vi "Dashboard Main - Copy (3).vi"() -> ()   [LabVIEW 2014]
uses:
  <vilib>/event_ctls.llb/eventvkey.ctl
  <vilib>/Rock Robotics/WPI/Dashboard/WPI_DashboardLogging Global.vi
  <vilib>/Utility/config.llb/Write Key (String).vi
  <vilib>/Utility/config.llb/Write Key (I32).vi
  <vilib>/Utility/config.llb/NI_LVConfig.lvlib
panel:
  in  "TCP":refnum<k5>
  in  "Rec Mode":enum32{"Stop", "Record", "Playback"}(radio)
  in  "Vision":u16(ring) items=["Camera Off", "USB Camera SW", "USB Camera HW", "IP Camera"]
  out "Camera IP":string
  out "Image Message":string="Timeout in Camera Communications"
  in  "Dashboard Tab":T1(tab)
  out "Low Battery":bool
  out "FMS":bool
  out "Teleop Mode":bool
  out "Auto Mode":bool
  out "Disabled":bool
  in  "Program":string
  in  "Camera Settings":T2={"Frame Rate"=30, "Compression"=30, "Size"=1} {"Frame Rate" scale=1.0..30.0; "Size" items=["640x480", "320x240", "160x120"]}
  out "Mode":T3(ring)=enum."Auto Disabled"
  in  "DB Camera Config":bool
  out "fps":dbl format="%#.1g"
  out "Mbps":dbl format="%#.1g"
  out "Mbps 2":bool
  in  "LCD_Line_10":string caption="DB/String 0"
  in  "LCD_Line_9":string caption="DB/String 0"
  in  "LCD_Line_8":string caption="DB/String 0"
  in  "LCD_Line_7":string caption="DB/String 0"
  in  "LCD_Line_6":string caption="DB/String 0"
  in  "LCD_Line_5":string caption="DB/String 0"
  in  "LCD_Line_4":string caption="DB/String 0"
  in  "LCD_Line_3":string caption="DB/String 0"
  in  "LCD_Line_2":string caption="DB/String 0"
  in  "LCD_Line_1":string caption="DB/String 0"
  in  "DB/String 9":string
  in  "DB/String 8":string
  in  "DB/String 7":string
  in  "DB/String 6":string
  in  "DB/String 5":string
  in  "DB/String 4":string
  in  "DB/String 3":string
  in  "DB/String 2":string
  in  "DB/String 1":string
  in  "DB/String 0":string
  in  "DB/Slider 0":dbl(slide) scale=0.0..5.0
  in  "DB/Slider 1":dbl(slide) scale=0.0..5.0
  in  "DB/Slider 2":dbl(slide) scale=0.0..5.0
  in  "DB/Slider 3":dbl(slide) scale=0.0..5.0
  out "DB/LED 3":bool
  out "DB/LED 2":bool
  out "DB/LED 1":bool
  out "DB/LED 0":bool
  in  "DB/Button 3":bool
  in  "DB/Button 2":bool
  in  "DB/Button 1":bool
  in  "DB/Button 0":bool caption="New Name"
  in  "Test Slider":dbl(slide) scale=0.0..100.0 scale format="%#_3g"
  in  "On/Off":bool caption="Solenoid"
  in  "Test Name":u16(ring) items=["Select the test to run...", "Example Test", "-------------------------------", "List of tests is built in robot code.", "Replace with your own automated tests."]
  in  "Test Tree":string(tree)
  in  "Motor":cluster{"Value":dbl, "Enable":bool} {"Value" scale=-1.0..1.0 scale format="%#_3g"}
  out "Progress":T4 {"Test Progress" scale=0.0..100.0}
  in  "Rev/Fwd":cluster{"Forward":bool, "Reverse":bool}
  in  "Test Ring":u16(ring) items=["Monochrome", "Color"]
  in  "Listbox":i32(listbox)
  out "Tree":string(tree)
  out "Camera Image":T5(plugin-control)
  out "Boolean":bool
  # "Program:"
  # "Dashboard: 2015-02"
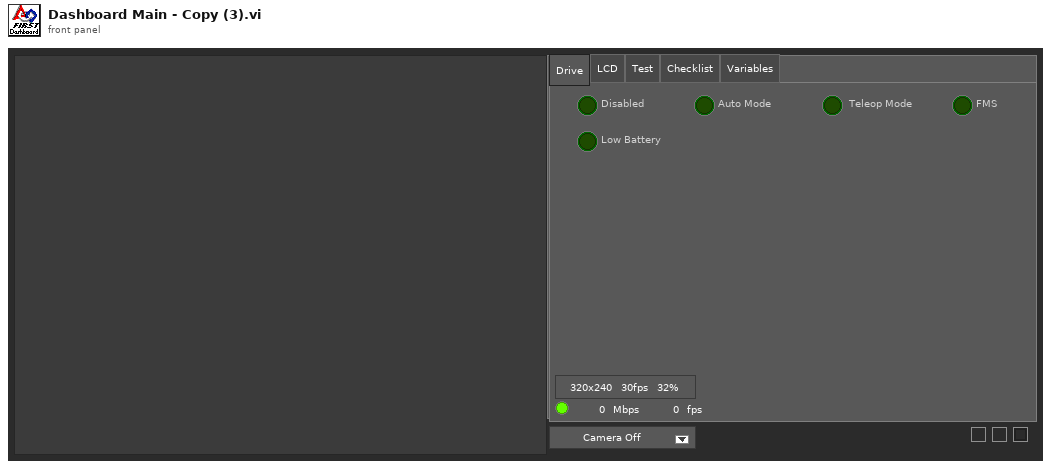
[diagram p1: front panel]
types:
  T1 = enum32{"Drive", "LCD", "Basic", "Test", "Checklist", "Variables"}
  T2 = cluster{"Frame Rate":i32, "Compression":i32, "Size":u16}
  T3 = enum8{"Tele-Op Disabled", "Tele-Op Enabled", "Auto Disabled", "Auto Enabled", "Test Disabled", "Test Enabled", "Disconnected", "No Code", "E-Stop"}
  T4 = cluster{"Test Progress":u8, "Test Progress Text":string}
  T5 = typedef "IMAQ Image.ctl" = refnum<image>
  T6 = enum32{"Drive", "Basic", "Custom", "Test", "Checklist", "Variables"}
  T7 = typedef "Image Type" = u32
  T8 = cluster{"Camera Image":refnum<vi>, "Dashboard Tab":refnum<vi>, "Boolean":refnum<vi>, "Vision":refnum<vi>, "Rec Mode":refnum<vi>, "Test Slider":refnum<vi>, "On/Off ":refnum<vi>, "Test Ring":refnum<vi>, "Rev/Fwd":refnum<vi>, "Test Name":refnum<vi>, "Motor":refnum<vi>, "Progress":refnum<vi>, "CheckList":refnum<vi>, "Tree":refnum<vi>, "Test Tree":refnum<vi>}
  T9 = cluster{"Error Strings":string, "Disable Counts":cluster{u16, u16}, "Rail Faults":cluster{u16, u16, u16}, "Robot IP":string, "DB Mode":u8, "Event Info":cluster{"Name":string, "Type":u8, "Number":u16, "Replay":u8}, "Camera Addr":string}
  T10 = cluster{"Storage":cluster{"Disk Free":u64, "RAM Block":u32, "RAM free":u32}, "CPU Utilization":cluster{"CPU % ISR":sgl, "CPU % Time Crit":sgl, "CPU % Timed Str":sgl, "CPU % High":sgl, "CPU % Above":sgl, "CPU % Normal":sgl, "CPU % Low":sgl}, "CAN":cluster{"% Bus Utilization":sgl, "Bus Off Cnt":u32, "TX_FIFO Full Cnt":u32, "Receive Error Cnt":u8, "Transmit Error Cnt":u8}, "HID":cluster{"HID Outputs":u32, "Rumble Low":u16, "Rumble High":u16}[]}
  T11 = cluster{"Status bits":cluster{"Test Mode":bool, "Autonomous":bool, "Enabled":bool, "Code Start":bool, "Brownout":bool, "Reserved 2":bool, "Reserved 3":bool, "E-Stop":bool}, "Code Trace":cluster{"Disabled":bool, "TeleOp":bool, "Auto":bool, "Test":bool}, "Controller Type":enum16{"unknown", "cRIO", "roboRio"}, "Code?":enum16{"unknown", "noCode", "code"}, "Battery V":dbl}
  T12 = cluster{"Control Bits":cluster{"TestMode":bool, "Autonomous":bool, "Enabled":bool, "FMS Present":bool, bool, bool, bool, "E-Stop":bool}, "Team Station ":u8, "Countdown":sgl, "Joystick Values":cluster{"Axes":dbl[], "Buttons":bool[], "POVs":i16[]}[]}
  T13 = cluster{"Axes":dbl[], "Buttons":bool[], "POVs":i16[]}[]
  T14 = cluster{"Axes":dbl[], "Buttons":bool[], "POVs":i16[]}
  T15 = typedef "NI_LVConfig.lvlib/Config Data RefNum.ctl" = refnum<k1>
  T16 = cluster{"Operation":enum16{"Update", "Clear"}, "Color Box":u32}[]
  T17 = typedef "eventvkey.ctl" = enum16{"ASCII", "Enter", "Return", "Shift", "Ctrl", "Alt", "Cmd", "Opt", "Caps", "NumLock", "Clear", "Break", "Up", "Down", "Left", "Right", "Insert", "Delete", "Home", "End", "PageUp", "PageDown", "Escape", "Help", "Pause", "ScrollLock", "F1", "F2", "F3", "F4", "F5", "F6", "F7", "F8", "F9", "F10", "F11", "F12", "F13", "F14", "F15", "F16", "F17", "F18", "F19", "F20", "F21", "F22", "F23", "F24", "Play", "VolumeUp", "VolumeDown", "Mute", "Two Byte Char"}
  T18 = cluster{"Image Size":bool, "Image Type":bool, "Pixel Value":bool, "ROI Information":bool, "Zoom Factor":bool}
  T19 = enum8{"Enabled", "Disabled", "Disabled and Grayed Out"}
  T20 = cluster{"Operation":enum16{"Update", "Clear"}, "Color Box":u32}
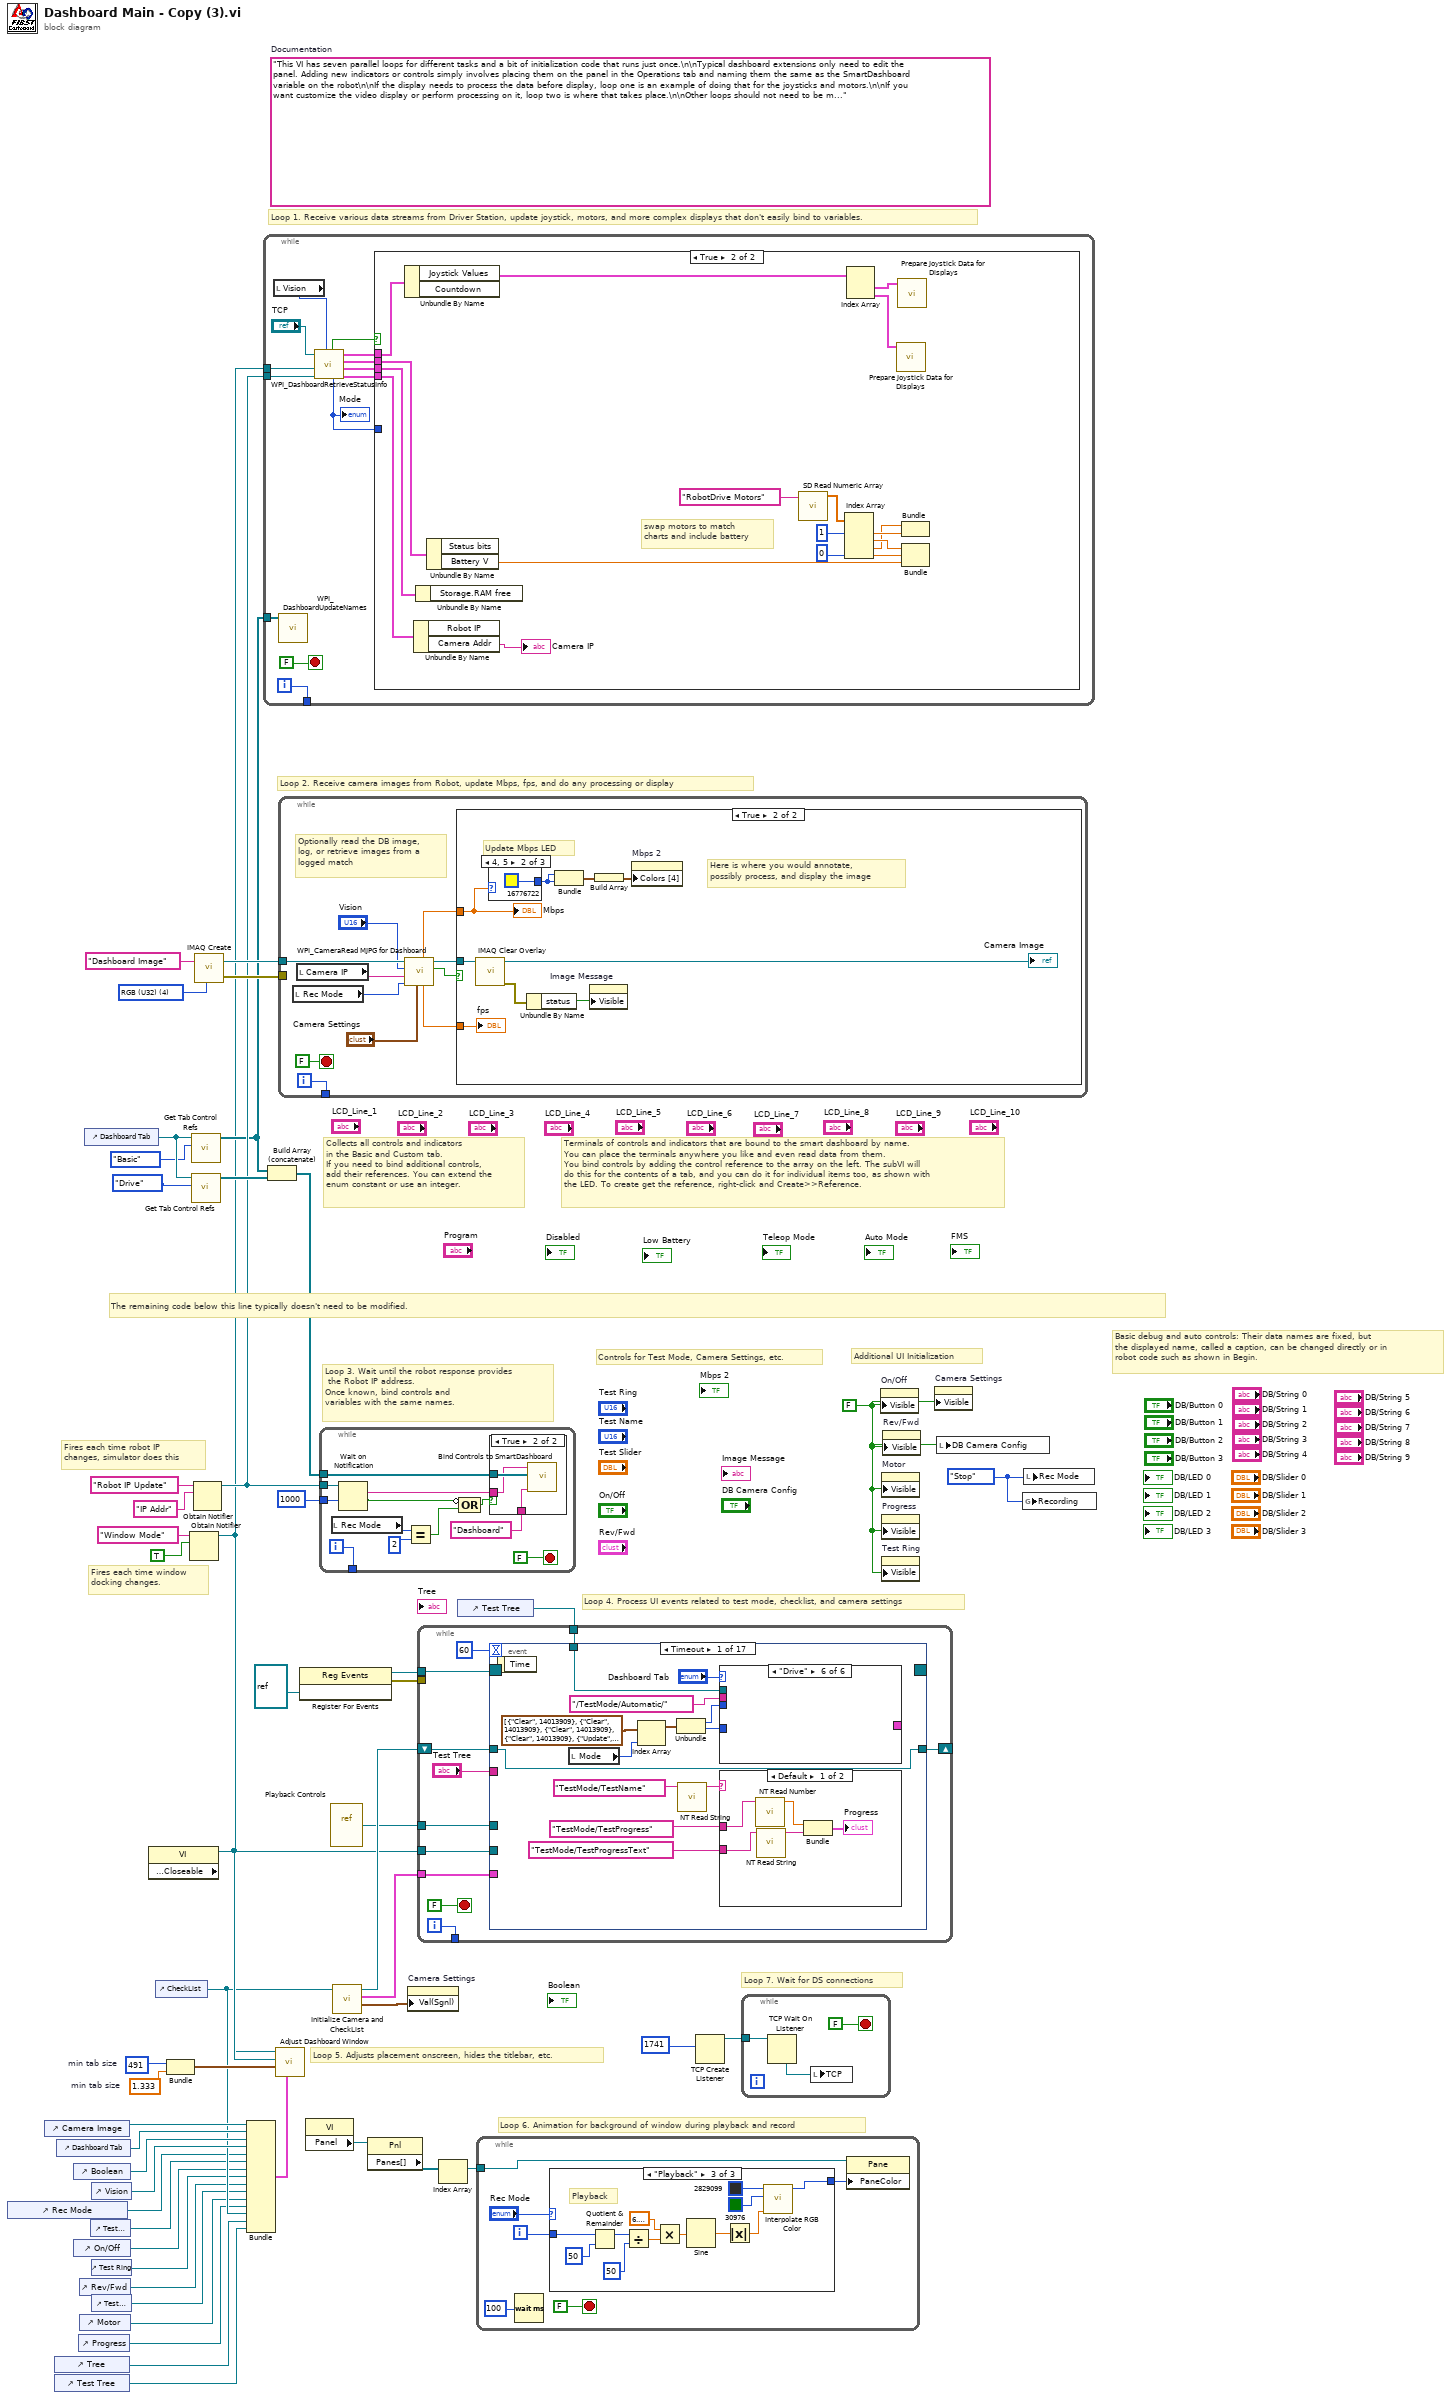
[diagram p0: block diagram]
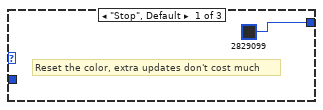
[diagram p3: hidden frame]
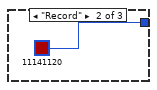
[diagram p4: hidden frame]
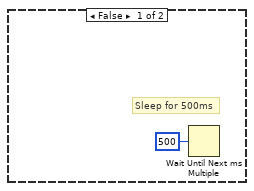
[diagram p6: hidden frame]
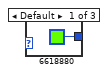
[diagram p7: hidden frame]
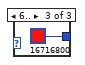
[diagram p8: hidden frame]
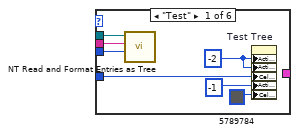
[diagram p9: hidden frame]
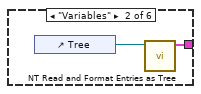
[diagram p10: hidden frame]
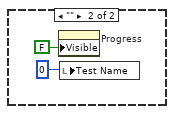
[diagram p14: hidden frame]
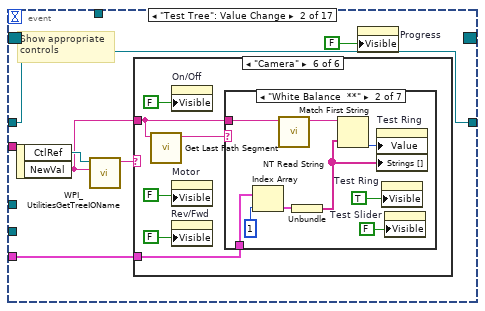
[diagram p15: hidden frame]
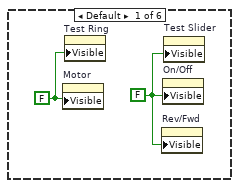
[diagram p16: hidden frame]
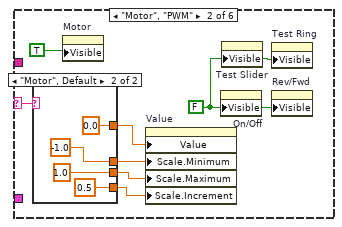
[diagram p17: hidden frame]
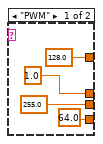
[diagram p18: hidden frame]
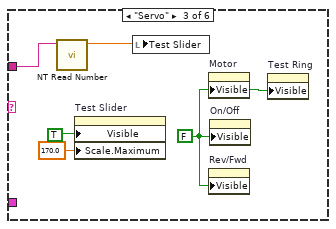
[diagram p19: hidden frame]
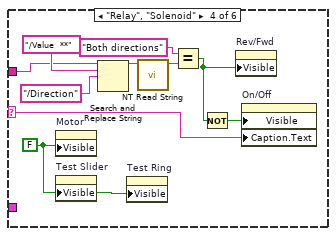
[diagram p20: hidden frame]
diagram:
  w24 = 491  # min tab size
  w23 = 1.333  # min tab size
  w32 = enum32{"Stop", "Record", "Playback"}."Stop" ("Rec Mode")
  w6 = FALSE ("Visible")
  (unwired) "This VI has seven parallel loops for different tasks and a bit of initialization code that runs just once.\n\nTypical dashboard extensions only need to edit the panel. Adding new indicators or controls simply involves placing them on the panel in the Operations tab and naming them the same as the SmartDashboard variable on the robot\n\nIf the display needs to process the data before display, loop one is an example of doing that for the joysticks and motors.\n\nIf you want customize the video display or perform processing on it, loop two is where that takes place.\n\nOther loops should not need to be modified. They are pretty standard, and document the task they perform."  # Documentation
  w52 = T7 4 items=["Grayscale (U8)", "Grayscale (I16)", "Grayscale (SGL)", "Complex (CSG)", "RGB (U32)", "HSL (U32)", "RGB (U64)"] ("Image Type")
  # "Loop 7. Wait for DS connections"
  # "Basic debug and auto controls: Their data names are fixed, but\nthe displayed name, called a caption, can be changed directly or in\nrobot code such as shown in Begin."
  # "Controls for Test Mode, Camera Settings, etc."
  # "Additional UI Initialization"
  # "Loop 6. Animation for background of window during playback and record"
  # "Fires each time robot IP\nchanges, simulator does this"
  # "Fires each time window\ndocking changes."
  # "Collects all controls and indicators\nin the Basic and Custom tab.\nIf you need to bind additional controls,\nadd their references. You can extend the\nenum constant or use an integer."
  # "The remaining code below this line typically doesn't need to be modified."
  # "Loop 4. Process UI events related to test mode, checklist, and camera settings"
  # "Terminals of controls and indicators that are bound to the smart dashboard by name.\nYou can place the terminals anywhere you like and even read data from them.\nYou bind controls by adding the control reference to the array on the left. The subVI will\ndo this for the contents of a tab, and you can do it for individual items too, as shown with\nthe LED. To create get the reference, right-click and Create>>Reference."
  # "Loop 3. Wait until the robot response provides\n the Robot IP address.\nOnce known, bind controls and\nvariables with the same names."
  # "Loop 5. Adjusts placement onscreen, hides the titlebar, etc."
  # "Loop 1. Receive various data streams from Driver Station, update joystick, motors, and more complex displays that don't easily bind to variables."
  # "Loop 2. Receive camera images from Robot, update Mbps, fps, and do any processing or display"
  n1 = control-ref of="Rec Mode"() -> (w12:refnum<vi>)
  n2 = control-ref of="Camera Image"() -> (w27:refnum<vi>)
  n3 = control-ref of="Tree"() -> (w16:refnum<vi>)
  n4 = control-ref of="Test Tree"() -> (w15:refnum<vi>)
  n5 = control-ref of="Dashboard Tab"() -> (w26:refnum<vi>)
  n6 = control-ref of="Boolean"() -> (w21:refnum<vi>)
  n7 = control-ref of="On/Off"() -> (w10:refnum<vi>)
  n8 = control-ref of="Progress"() -> (w7:refnum<vi>)
  n9 = control-ref of="Rev/Fwd"() -> (w8:refnum<vi>)
  n10 = control-ref of="Motor"() -> (w13:refnum<vi>)
  n11 = control-ref of="Dashboard Tab"() -> (w30:refnum<vi>)
  n12 = control-ref of="Test Slider"() -> (w11:refnum<vi>)
  n13 = control-ref of="Vision"() -> (w25:refnum<vi>)
  n14 = control-ref of="Test Ring"() -> (w9:refnum<vi>)
  n15 = control-ref of="Test Name"() -> (w14:refnum<vi>)
  n16 = property class="VI" props=["Front Panel.Closeable"]() -> (reference out=w31:refnum<vi>)  [unwired: 2 in, 2 out]
  n17 = control-ref of="CheckList"() -> (w17:refnum<vi>)
  n18 = Bundle("min tab size"=w24, "min tab size"=w23) -> (w22:cluster{"min tab size":i32, "min tab size":dbl})  [unwired: 1 in]
  n19 = Obtain Notifier(name (unnamed)="Window Mode", notification data type=TRUE) -> (notifier out=w3:refnum<notifier>)  [unwired: 2 in, 2 out]
  n20 = call <vilib>:"Get Tab Control Refs.vi"("Page Index"=T6."Basic" ("Dashboard Tab"), "TabControl in"=w30) -> ("ControlsOnPage"=w4:refnum<vi>[])  [unwired: 9 in]
  n21 = call <vilib>:"Get Tab Control Refs.vi"("Page Index"=T6."Drive" ("Dashboard Tab"), "TabControl in"=w30) -> ("ControlsOnPage"=w29:refnum<vi>[])  [unwired: 9 in]
  n22 = Obtain Notifier(name (unnamed)="Robot IP Update", notification data type="IP Addr" ("name (unnamed)")) -> (notifier out=w5:refnum<notifier>)  [unwired: 2 in, 2 out]
  n23 = call "IMAQ Create"("Image Name"="Dashboard Image", "Image Type"=w52) -> ("New Image"=w50:T5, "error out"=w49:errorcluster)  [unwired: 2 in, 1 out]
  n24 = Bundle("Camera Image"=w27, "Dashboard Tab"=w26, "Boolean"=w21, "Vision"=w25, "Rec Mode"=w12, "Test Slider"=w11, "On/Off"=w10, "Test Ring"=w9, "Rev/Fwd"=w8, "Test Name"=w14, "Motor"=w13, "Progress"=w7, "CheckList"=w17, "Tree"=w16, "Test Tree"=w15) -> (w18:T8)  [unwired: 1 in]
  n25 = while {
    tunnel: [w64] -> _
    tunnel: w5 -> [w58]
    tunnel: w4 -> [w57]
    tunnel: w3 -> [w53]
    i -> [w64]
    stop <- FALSE stop-if-true
    n26 = local read "Vision"() -> (w55:u16)
    n27 = call <vilib>:"WPI_DashboardUpdateNames.vi"("Controls on Tab"=w57) -> ()  [unwired: 11 in]
    n28 = call <vilib>:"WPI_DashboardRetrieveStatusInfo.vi"("Vision"=w55, "Binding Refnum"=w58, "Window Mode Notifier"=w53, "TCP Cnx"="TCP") -> ("Power and Errors"=w59:T9, "Robot Metrics"=w62:T10, "Status Info"=w63:T11, "Control Info"=w60:T12, "Robot Mode"=w56:T3, "Process?"=w61:bool)  [unwired: 2 in]
    "Mode" <- w56
    n29 = case shown="True" w61 {
      tunnel: w63 -> [_ w82]
      tunnel: w62 -> [_ w81]
      tunnel: w60 -> [_ w80]
      tunnel: w59 -> [_ w79]
      tunnel: w56 -> [_ _]
      frame False {
      }
      frame True {
        # "swap motors to match\ncharts and include battery"
        n30 = Unbundle By Name(w80) -> ("Joystick Values"=w69:T13)  [unwired: 1 out]
        n31 = Unbundle By Name(w79) -> ("Camera Addr"=→"Camera IP":string)  [unwired: 1 out]
        n32 = Unbundle By Name(w81) -> ()  [unwired: 1 out]
        n33 = Unbundle By Name(w82) -> ("Battery V"=w70:dbl)  [unwired: 1 out]
        n34 = call <vilib>:"SD Read Numeric Array.vi"("Name"="RobotDrive Motors") -> ("Numeric Array"=w72:dbl[])  [unwired: 8 in, 2 out]
        n35 = Index Array(array=w72, index #1=1, index #4=0) -> (element #1=w74:dbl, element #2=w75:dbl, element #3=w73:dbl, element #4=w78:dbl)  [unwired: 2 in]
        n36 = Index Array(array=w69) -> (element #1=w68:T14, element #2=w66:T14)  [unwired: 2 in]
        n37 = call "Prepare Joystick Data for Displays.vi"("Joystick Values"=w66) -> ()  [unwired: 8 in, 3 out]
        n38 = call "Prepare Joystick Data for Displays.vi"("Joystick Values"=w68) -> ()  [unwired: 8 in, 3 out]
        n39 = Bundle("Numeric"=w73, "Numeric"=w74) -> ()  [unwired: 1 in, 1 out]
        n40 = Bundle("Numeric"=w75, "Numeric"=w78, "Battery V"=w70) -> ()  [unwired: 1 in, 1 out]
      }
    }
  }
  n41 = Build Array (concatenate)(w4, w29) -> (w28:refnum<vi>[])
  n42 = call "Adjust Dashboard Window.vi"("Sizing Refnums"=w18, "Size Constraints"=w22, "VI"=w31, "Notifier in"=w3) -> ()  [unwired: 8 in]
  n43 = while {
    tunnel: w50 -> [w91]
    tunnel: w49 -> [_]
    tunnel: [w92] -> _
    i -> [w92]
    stop <- FALSE stop-if-true
    # "Optionally read the DB image,\nlog, or retrieve images from a\nlogged match"
    n44 = local read "Rec Mode"() -> (w85:enum32{"Stop", "Record", "Playback"})
    n45 = local read "Camera IP"() -> (w83:string)
    n46 = call <vilib>:"WPI_CameraRead MJPG for Dashboard.vi"("Camera Settings"="Camera Settings", "Rec Mode"=w85, "Camera IP"=w83, "Camera Mode"="Vision", "Refnum in"=w91) -> ("Active"=w89:bool, "Refnum out"=w90:T5, "FPS"=w88:dbl, "Bandwidth (Mbps)"=w87:dbl)  [unwired: 3 in]
    n47 = case shown="True" w89 {
      tunnel: w90 -> [_ w98]
      tunnel: w87 -> [_ w97]
      tunnel: w88 -> [_ w95]
      frame False {
        # "Sleep for 500ms"
        n48 = Wait Until Next ms Multiple(millisecond multiple=u32 500) -> ()  [unwired: 1 out]
      }
      frame True {
        # "Here is where you would annotate,\npossibly process, and display the image"
        # "Update Mbps LED"
        n49 = call "IMAQ Clear Overlay"("Image"=w98) -> ("error out"=w102:errorcluster, "Image Out"=→"Camera Image":T5)  [unwired: 2 in, 7 out]
        n50 = case shown="4, 5" w97 {
          tunnel: [u32 6618880 ("Color Box") u32 16776722 ("Color Box") u32 16716800 ("Color Box")] -> w99
          frame Default {
          }
          frame 4, 5 {
          }
          frame 6.. {
          }
        }
        n51 = Unbundle By Name(w102) -> ("status"=w103:bool)
        n52 = Bundle("Color Box"=w99, "Color Box"=w99) -> (w101:cluster{"Color Box":u32, "Color Box":u32})  [unwired: 1 out]
        n53 = property on="Image Message" class="Str"("Visible"=w103) -> ()  [unwired: 2 in, 2 out]
        n54 = Build Array(w101) -> (w100:cluster{"Color Box":u32, "Color Box":u32}[])
        n55 = property on="Mbps 2" class="Bool (strict)"("Colors [4]"=w100) -> ()  [unwired: 2 in, 2 out]
        "Mbps" <- w97
        "fps" <- w95
      }
    }
  }
  n56 = register-events(refnum<vi> refnum) -> (reference out=w36:refnum<event-registration>, error out=w35:errorcluster)  [unwired: 2 in]
  n57 = property class="VI"() -> ("Panel"=w39:refnum<vi>)  [unwired: 2 in, 2 out]
  n58 = while {
    tunnel: w28 -> [w118]
    tunnel: w5 -> [w116]
    tunnel: [w114] -> _
    tunnel: u32 1000 ("milliseconds to wait") -> [w113]
    i -> [w114]
    stop <- FALSE stop-if-true
    n59 = local read "Rec Mode"() -> (w109:enum32{"Stop", "Record", "Playback"})
    n60 = Wait on Notification(notifier=w116, timeout in ms (-1)=w113) -> (notification=w115:string, timed out?=w111:bool)  [unwired: 2 in, 2 out]
    n61 = Equal?(x=w109, y=u16 2 ("Rec Mode")) -> (x = y?=w110:bool)
    n62 = Compound Arithmetic op=OR(invert w111, w110) -> (w112:bool)
    n63 = case shown="True" w112 {
      tunnel: w118 -> [_ w121]
      tunnel: w115 -> [_ w120]
      tunnel: "Dashboard" -> [_ w119]
      frame False {
      }
      frame True {
        n64 = call <vilib>:"Bind Controls to SmartDashboard.vi"("Client Name"=w119, "Bound Control Refs"=w121, "Server IP Address"=w120) -> ()  [unwired: 9 in]
      }
    }
  }
  n65 = vi-ref "Playback Controls.vi"() -> (w37:refnum<vi>)
  n66 = call "Initialize Camera and CheckList.vi"("ListBox in"=w17) -> ("Cluster"=w43:cluster{"value":i32, "value":i32, "index":i32}, "Array"=w44:cluster{string[]}[], "File Refnum"=w42:T15)  [unwired: 8 in]
  n67 = property class="Pnl"(reference=w39) -> ("Panes[]"=w40:refnum<vi>[])  [unwired: 1 in, 2 out]
  n68 = property on="Camera Settings" class="Clust (strict)"("Val(Sgnl)"=w43) -> ()  [unwired: 2 in, 2 out]
  n69 = Index Array(array=w40) -> (element=w38:refnum<vi>)  [unwired: 1 in]
  n70 = control-ref of="Test Tree"() -> (w41:refnum<vi>)
  n71 = while {
    tunnel: w44 -> [w129]
    shift-right: [w128] -> _
    shift-left: w42 -> [w127]
    tunnel: [w126] -> _
    tunnel: w41 -> [w125]
    tunnel: w37 -> [w124]
    tunnel: w36 -> [w123]
    tunnel: w35 -> [_]
    tunnel: w31 -> [w122]
    i -> [w126]
    stop <- FALSE stop-if-true
    n72 = event shown="[0] Timeout" {
      selector: w123 -> [_ _ _ _ _ _ _ _ _ _ _ _ _ _ _ _ _]
      dyn-events: [_ _ _ _ _ _ _ _ _ _ _ _ _ w367 _ _ _] -> _
      timeout: u32 60 ("milliseconds to wait") -> [_ _ _ _ _ _ _ _ _ _ _ _ _ _ _ _ _]
      tunnel: w125 -> [w141 _ _ _ _ _ _ _ _ _ _ _ _ _ _ _ _]
      tunnel: "Test Tree" -> [_ _ _ _ _ _ _ _ w336 w344 w346 w350 w358 _ _ _ _]
      tunnel: w129 -> [_ w163 _ _ _ _ w300 w330 _ _ _ _ _ _ _ _ _]
      tunnel: [w137 w162 w261 w266 w274 w286 w299 w323 w335 w342 w345 w349 w357 w369 w383 w384 w394] -> w128
      tunnel: w127 -> [w137 w162 w261 w266 w274 w286 w298 w323 w335 w342 w345 w349 w357 w369 w383 w384 w394]
      tunnel: w124 -> [_ _ _ _ _ _ _ _ _ _ _ _ _ w370 _ w387 _]
      tunnel: w122 -> [_ _ _ _ _ _ _ _ _ _ _ _ _ w365 _ _ _]
      event Timeout {
        n73 = event-data() -> ()  [unwired: 1 in, 1 out]
        n74 = local read "Mode"() -> (w140:T3)
        n75 = Index Array(array=T16 [{"Operation"=enum."Clear", "Color Box"=14013909}, {"Operation"=enum."Clear", "Color Box"=14013909}, {"Operation"=enum."Clear", "Color Box"=14013909}, {"Operation"=enum."Clear", "Color Box"=14013909}, {"Operation"=enum."Update", "Color Box"=14013909}, {"Operation"=enum."Update", "Color Box"=16777215}, {"Operation"=enum."Clear", "Color Box"=14013909}, {"Operation"=enum."Clear", "Color Box"=14013909}, {"Operation"=enum."Clear", "Color Box"=14013909}], index=w140) -> (element=w135:T20)
        n76 = Unbundle(w135) -> ("Operation"=w134:enum16{"Update", "Clear"}, "Color Box"=w133:u32)
        n77 = call <vilib>:"NT Read String.vi"("Name"="TestMode/TestName") -> ("String"=w144:string)  [unwired: 9 in, 1 out]
        n78 = case shown="\"Drive\"" "Dashboard Tab" {
          tunnel: w141 -> [w152 _ _ _ _ _]
          tunnel: "/TestMode/Automatic/" ("Name Pattern") -> [w151 _ _ _ _ _]
          tunnel: w134 -> [w150 _ _ _ _ _]
          tunnel: [_ w154 _ _ _ _] -> _
          tunnel: w133 -> [w146 _ _ _ _ _]
          frame "Test" {
            w149 = -2 ("Active Item:Row Number")
            n79 = call <vilib>:"NT Read and Format Entries as Tree.vi"("Operation"=w150, "Name Pattern"=w151, "Tree Refnum"=w152) -> ()  [unwired: 7 in, 2 out]
            n80 = property on="Test Tree" class="Tree (strict)"("Active Item Row Number"=w149, "ActiveColNum"=w149, "CellBG"=w146, "Active Item Row Number"=-1 ("Active Item:Row Number"), "CellBG"=u32 5789784 ("Color Box")) -> ()  [unwired: 2 in, 2 out]
          }
          frame "Variables" {
            n81 = control-ref of="Tree"() -> (w153:refnum<vi>)
            n82 = call <vilib>:"NT Read and Format Entries as Tree.vi"("Tree Refnum"=w153) -> ("Formatted Strings"=w154:cluster{"Name":string, "Value":string}[])  [unwired: 9 in, 1 out]
          }
          frame "Checklist" {
          }
          frame "Basic" {
          }
          frame "LCD" {
          }
          frame "Drive" {
          }
        }
        n83 = case shown="Default" w144 {
          tunnel: "TestMode/TestProgress" ("Name") -> [w156 _]
          tunnel: "TestMode/TestProgressText" ("Name") -> [w155 _]
          frame Default {
            n84 = call <vilib>:"NT Read Number.vi"("Name"=w156) -> ("Numeric"=w157:dbl)  [unwired: 9 in, 1 out]
            n85 = call <vilib>:"NT Read String.vi"("Name"=w155) -> ("String"=w158:string)  [unwired: 9 in, 1 out]
            n86 = Bundle("Numeric"=w157, "String"=w158) -> (→"Progress":cluster{"Numeric":dbl, "String":string})  [unwired: 1 in]
          }
          frame "" {
            n87 = property on="Progress" class="Clust (strict)"("Visible"=FALSE) -> ()  [unwired: 2 in, 2 out]
            n88 = local write "Test Name"(u16 0) -> ()
          }
        }
      }
      event "Test Tree": Value Change {
        # "Show appropriate\ncontrols"
        n89 = event-data() -> ("CtlRef"=w166:refnum<vi>, "NewVal"=w164:string)  [unwired: 1 in]
        n90 = call <vilib>:"WPI_UtilitiesGetTreeIOName.vi"("NewVal"=w164, "TreeControl in"=w166) -> ("I/O Name"=w167:string)  [unwired: 9 in]
        n91 = case shown="\"Camera\"" w167 {
          selector: w167 -> [_ w174 _ w192 w201 _]
          tunnel: w164 -> [_ _ w189 w191 _ w208]
          tunnel: w163 -> [_ _ _ _ _ w207]
          frame Default {
            w169 = FALSE ("Visible")
            w168 = FALSE ("Visible")
            n92 = property on="Motor" class="Clust (strict)"("Visible"=w168) -> ()  [unwired: 2 in, 2 out]
            n93 = property on="Test Ring" class="Ring (strict)"("Visible"=w168) -> ()  [unwired: 2 in, 2 out]
            n94 = property on="Rev/Fwd" class="Clust (strict)"("Visible"=w169) -> ()  [unwired: 2 in, 2 out]
            n95 = property on="On/Off" class="Bool (strict)"("Visible"=w169) -> ()  [unwired: 2 in, 2 out]
            n96 = property on="Test Slider" class="Slide (strict)"("Visible"=w169) -> ()  [unwired: 2 in, 2 out]
          }
          frame "Motor", "PWM" {
            w175 = FALSE ("Visible")
            n97 = case shown="\"Motor\", Default" w174 {
              tunnel: [1.0 ("Value") -1.0 ("Value")] -> w173
              tunnel: [255.0 ("Value") 1.0 ("Value")] -> w172
              tunnel: [128.0 ("Value") 0.0 ("Value")] -> w171
              tunnel: [64.0 ("Value") 0.5 ("Value")] -> w170
              frame "PWM" {
              }
              frame "Motor", Default {
              }
            }
            n98 = property on="Motor" class="Clust (strict)"("Visible"=TRUE) -> ()  [unwired: 2 in, 2 out]
            n99 = property on="Value" class="Slide (strict)"("Value"=w171, "Scale.Minimum"=w173, "Scale.Maximum"=w172, "Scale.Increment"=w170) -> ()  [unwired: 2 in, 2 out]
            n100 = property on="On/Off" class="Bool (strict)"("Visible"=w175) -> ()  [unwired: 2 in, 2 out]
            n101 = property on="Test Slider" class="Slide (strict)"("Visible"=w175) -> ()  [unwired: 2 in, 2 out]
            n102 = property on="Test Ring" class="Ring (strict)"("Visible"=w175) -> ()  [unwired: 2 in, 2 out]
            n103 = property on="Rev/Fwd" class="Clust (strict)"("Visible"=w175) -> ()  [unwired: 2 in, 2 out]
          }
          frame "Servo" {
            w187 = FALSE ("Visible")
            n104 = call <vilib>:"NT Read Number.vi"("Name"=w189) -> ("Numeric"=w188:dbl)  [unwired: 9 in, 1 out]
            n105 = property on="Test Slider" class="Slide (strict)"("Visible"=TRUE, "Scale.Maximum"=170.0 ("Scale.Range:Maximum")) -> ()  [unwired: 2 in, 2 out]
            n106 = local write "Test Slider"(w188) -> ()
            n107 = property on="Motor" class="Clust (strict)"("Visible"=w187) -> ()  [unwired: 2 in, 2 out]
            n108 = property on="Rev/Fwd" class="Clust (strict)"("Visible"=w187) -> ()  [unwired: 2 in, 2 out]
            n109 = property on="On/Off" class="Bool (strict)"("Visible"=w187) -> ()  [unwired: 2 in, 2 out]
            n110 = property on="Test Ring" class="Ring (strict)"("Visible"=w187) -> ()  [unwired: 2 in, 2 out]
          }
          frame "Relay", "Solenoid" {
            w190 = FALSE ("Visible")
            n111 = property on="Motor" class="Clust (strict)"("Visible"=w190) -> ()  [unwired: 2 in, 2 out]
            n112 = property on="Test Slider" class="Slide (strict)"("Visible"=w190) -> ()  [unwired: 2 in, 2 out]
            n113 = Search and Replace String(input string=w191, search string="/Value  **", replace string="/Direction") -> (result string=w197:string)  [unwired: 5 in, 3 out]
            n114 = property on="Test Ring" class="Ring (strict)"("Visible"=w190) -> ()  [unwired: 2 in, 2 out]
            n115 = call <vilib>:"NT Read String.vi"("Name"=w197) -> ("String"=w195:string)  [unwired: 9 in, 1 out]
            n116 = Equal?(x="Both directions", y=w195) -> (x = y?=w193:bool)
            n117 = Not(x=w193) -> (.not. x?=w194:bool)
            n118 = property on="Rev/Fwd" class="Clust (strict)"("Visible"=w193) -> ()  [unwired: 2 in, 2 out]
            n119 = property on="On/Off" class="Bool (strict)"("Visible"=w194, "Caption.Text"=w192) -> ()  [unwired: 2 in, 2 out]
          }
          frame "Compressor", "Digital Out" {
            w200 = FALSE ("Visible")
            # "Get direction and finish"
            n120 = property on="Motor" class="Clust (strict)"("Visible"=w200) -> ()  [unwired: 2 in, 2 out]
            n121 = property on="Test Slider" class="Slide (strict)"("Visible"=w200) -> ()  [unwired: 2 in, 2 out]
            n122 = property on="Test Ring" class="Ring (strict)"("Visible"=w200) -> ()  [unwired: 2 in, 2 out]
            n123 = property on="On/Off" class="Bool (strict)"("Visible"=TRUE, "Caption.Text"=w201) -> ()  [unwired: 2 in, 2 out]
            n124 = property on="Rev/Fwd" class="Clust (strict)"("Visible"=FALSE) -> ()  [unwired: 2 in, 2 out]
          }
          frame "Camera" {
            n125 = call <vilib>:"Get Last Path Segment.vi"("String in"=w208) -> ("String out"=w209:string)  [unwired: 10 in]
            n126 = property on="On/Off" class="Bool (strict)"("Visible"=FALSE) -> ()  [unwired: 2 in, 2 out]
            n127 = property on="Motor" class="Clust (strict)"("Visible"=FALSE) -> ()  [unwired: 2 in, 2 out]
            n128 = property on="Rev/Fwd" class="Clust (strict)"("Visible"=FALSE) -> ()  [unwired: 2 in, 2 out]
            n129 = case shown="\"White Balance  **\"" w209 {
              tunnel: w208 -> [w215 w224 w233 w242 w251 _ w257]
              tunnel: w207 -> [w213 w221 w230 w239 w248 _ _]
              frame "Size  **" {
                n130 = Index Array(array=w213) -> (element=w212:cluster{string[]})  [unwired: 1 in]
                n131 = call <vilib>:"NT Read String.vi"("Name"=w215) -> ("String"=w214:string)  [unwired: 9 in, 1 out]
                n132 = Unbundle(w212) -> (w210:string[])
                n133 = Match First String(2:w210, 3:w214) -> (0:w211:i32)  [unwired: 1 out]
                n134 = property on="Test Ring" class="Ring (strict)"("Value"=w211, "Strings []"=w210) -> ()  [unwired: 2 in, 2 out]
                n135 = property on="Test Ring" class="Ring (strict)"("Visible"=TRUE) -> ()  [unwired: 2 in, 2 out]
                n136 = property on="Test Slider" class="Slide (strict)"("Visible"=FALSE) -> ()  [unwired: 2 in, 2 out]
              }
              frame "White Balance  **" {
                n137 = Index Array(array=w221, index=1) -> (element=w222:cluster{string[]})
                n138 = call <vilib>:"NT Read String.vi"("Name"=w224) -> ("String"=w223:string)  [unwired: 9 in, 1 out]
                n139 = Unbundle(w222) -> (w219:string[])
                n140 = Match First String(2:w219, 3:w223) -> (0:w218:i32)  [unwired: 1 out]
                n141 = property on="Test Ring" class="Ring (strict)"("Value"=w218, "Strings []"=w219) -> ()  [unwired: 2 in, 2 out]
                n142 = property on="Test Ring" class="Ring (strict)"("Visible"=TRUE) -> ()  [unwired: 2 in, 2 out]
                n143 = property on="Test Slider" class="Slide (strict)"("Visible"=FALSE) -> ()  [unwired: 2 in, 2 out]
              }
              frame "Exposure  **" {
                n144 = Index Array(array=w230, index=2) -> (element=w231:cluster{string[]})
                n145 = call <vilib>:"NT Read String.vi"("Name"=w233) -> ("String"=w232:string)  [unwired: 9 in, 1 out]
                n146 = Unbundle(w231) -> (w227:string[])
                n147 = Match First String(2:w227, 3:w232) -> (0:w228:i32)  [unwired: 1 out]
                n148 = property on="Test Ring" class="Ring (strict)"("Value"=w228, "Strings []"=w227) -> ()  [unwired: 2 in, 2 out]
                n149 = property on="Test Ring" class="Ring (strict)"("Visible"=TRUE) -> ()  [unwired: 2 in, 2 out]
                n150 = property on="Test Slider" class="Slide (strict)"("Visible"=FALSE) -> ()  [unwired: 2 in, 2 out]
              }
              frame "Exposure Priority  **" {
                n151 = Index Array(array=w239, index=3) -> (element=w240:cluster{string[]})
                n152 = call <vilib>:"NT Read String.vi"("Name"=w242) -> ("String"=w241:string)  [unwired: 9 in, 1 out]
                n153 = Unbundle(w240) -> (w236:string[])
                n154 = Match First String(2:w236, 3:w241) -> (0:w237:i32)  [unwired: 1 out]
                n155 = property on="Test Ring" class="Ring (strict)"("Value"=w237, "Strings []"=w236) -> ()  [unwired: 2 in, 2 out]
                n156 = property on="Test Ring" class="Ring (strict)"("Visible"=TRUE) -> ()  [unwired: 2 in, 2 out]
                n157 = property on="Test Slider" class="Slide (strict)"("Visible"=FALSE) -> ()  [unwired: 2 in, 2 out]
              }
              frame "Color Enable  **" {
                n158 = Index Array(array=w248, index=4) -> (element=w249:cluster{string[]})
                n159 = call <vilib>:"NT Read String.vi"("Name"=w251) -> ("String"=w250:string)  [unwired: 9 in, 1 out]
                n160 = Unbundle(w249) -> (w245:string[])
                n161 = Match First String(2:w245, 3:w250) -> (0:w246:i32)  [unwired: 1 out]
                n162 = property on="Test Ring" class="Ring (strict)"("Value"=w246, "Strings []"=w245) -> ()  [unwired: 2 in, 2 out]
                n163 = property on="Test Ring" class="Ring (strict)"("Visible"=TRUE) -> ()  [unwired: 2 in, 2 out]
                n164 = property on="Test Slider" class="Slide (strict)"("Visible"=FALSE) -> ()  [unwired: 2 in, 2 out]
              }
              frame Default {
                n165 = property on="Test Ring" class="Ring (strict)"("Visible"=FALSE) -> ()  [unwired: 2 in, 2 out]
                n166 = property on="Test Slider" class="Slide (strict)"("Visible"=FALSE) -> ()  [unwired: 2 in, 2 out]
              }
              frame "Brightness  **", "Color Level  **", "Compression  **", "FPS  **", "Sharpness  **" {
                n167 = call <vilib>:"NT Read Number.vi"("Name"=w257) -> ("Numeric"=w256:dbl)  [unwired: 9 in, 1 out]
                n168 = local write "Test Slider"(w256) -> ()
                n169 = property on="Test Slider" class="Slide (strict)"("Visible"=TRUE, "Scale.Maximum"=100.0 ("Scale.Range:Maximum")) -> ()  [unwired: 2 in, 2 out]
                n170 = property on="Test Ring" class="Ring (strict)"("Visible"=FALSE) -> ()  [unwired: 2 in, 2 out]
              }
            }
          }
        }
        n171 = property on="Progress" class="Clust (strict)"("Visible"=FALSE) -> ()  [unwired: 2 in, 2 out]
      }
      event "Test Name": Mouse Enter {
        # "Populate the ring with the list of tests"
        n172 = event-data() -> ()  [unwired: 1 in, 1 out]
        n173 = call <vilib>:"NT Read String Array.vi"("Name"="TestMode/TestList") -> ("String Array"=w265:string[])  [unwired: 9 in, 1 out]
        n174 = Build Array (concatenate)("Select the test to run...", w265) -> (w264:string[])
        n175 = property on="Test Name" class="Ring (strict)"("Strings []"=w264) -> ()  [unwired: 2 in, 2 out]
      }
      event "Test Name": Value Change {
        w267 = FALSE ("Visible")
        # "Tell the robot the test name to run"
        n176 = event-data() -> ("NewVal"=w271:u16)  [unwired: 1 in]
        n177 = property on="Test Name" class="Ring (strict)"() -> ("Strings []"=w272:string[])  [unwired: 2 in, 2 out]
        n178 = local write "Progress"(T4 {"Test Progress"=0, "Test Progress Text"=""} ("Progress")) -> ()
        n179 = Index Array(array=w272, index=w271) -> (element=w270:string)
        n180 = call <vilib>:"NT Write String.vi"("String"=w270, "Name"="TestMode/TestName") -> ()  [unwired: 9 in, 1 out]
        n181 = property on="Progress" class="Clust (strict)"("Visible"=TRUE) -> ()  [unwired: 2 in, 2 out]
        n182 = property on="Motor" class="Clust (strict)"("Visible"=w267) -> ()  [unwired: 2 in, 2 out]
        n183 = property on="Test Slider" class="Slide (strict)"("Visible"=w267) -> ()  [unwired: 2 in, 2 out]
        n184 = property on="On/Off" class="Bool (strict)"("Visible"=w267) -> ()  [unwired: 2 in, 2 out]
        n185 = property on="Rev/Fwd" class="Clust (strict)"("Visible"=w267) -> ()  [unwired: 2 in, 2 out]
        n186 = property on="Test Ring" class="Ring (strict)"("Visible"=w267) -> ()  [unwired: 2 in, 2 out]
      }
      event "Listbox": Double Click {
        # "Shift clears all"
        # "Update symbols on the listbox"
        n187 = event-data() -> ("PlatMods.Shift"=w275:bool, "Row"=w277:i32)  [unwired: 1 in]
        n188 = case shown="True" w275 {
          tunnel: w277 -> [w281 _]
          tunnel: 1 -> [w280 _]
          frame False {
            n189 = property on="Listbox" class="LstBox (strict)"() -> ("Item Symbols"=w279:i32[])  [unwired: 2 in, 2 out]
            n190 = Replace Array Subset(array=w279, new element=w280, index=w281) -> (w278:i32[])
            n191 = property on="Listbox" class="LstBox (strict)"("Item Symbols"=w278) -> ()  [unwired: 2 in, 2 out]
          }
          frame True {
            w282 = 0 ("Top Row")
            n192 = property on="Listbox" class="LstBox (strict)"() -> ("Number of Rows"=w284:u32)  [unwired: 2 in, 2 out]
            n193 = Initialize Array(0, w284) -> (w283:i32[])
            n194 = property on="Listbox" class="LstBox (strict)"("Top Row"=w282, "Value"=w282, "Item Symbols"=w283) -> ()  [unwired: 2 in, 2 out]
          }
        }
      }
      event "Listbox": Key Down {
        # "Update symbols on the listbox\nLeft and right keys check and uncheck"
        n195 = event-data() -> ("VKey"=w288:T17)  [unwired: 1 in]
        n196 = case shown="\"Left\", \"Right\"" w288 {
          selector: w288 -> [w293 _]
          tunnel: eventvkey."Left" ("VKey") -> [w291 _]
          frame "Left", "Right" {
            n197 = Equal?(x=w291, y=w293) -> (x = y?=w292:bool)
            n198 = Select(t=0, s=w292, f=1) -> (s? t:f=w294:i32)
            n199 = property on="Listbox" class="LstBox (strict)"() -> ("Item Symbols"=w297:i32[])  [unwired: 2 in, 2 out]
            n200 = Replace Array Subset(array=w297, new element=w294, index="Listbox") -> (w296:i32[])
            n201 = property on="Listbox" class="LstBox (strict)"("Item Symbols"=w296) -> ()  [unwired: 2 in, 2 out]
          }
          frame Default {
          }
        }
      }
      event "DB Camera Config": Value Change {
        # "Show or hide the cluster of controls, store in ini file"
        n202 = event-data() -> ("NewVal"=w301:bool)  [unwired: 1 in]
        n203 = case shown="False" w301 {
          tunnel: w300 -> [w310 _]
          tunnel: [w303 w321] -> w299
          tunnel: w298 -> [w302 w321]
          frame False {
            w317 = "Camera"
            w320 = FALSE ("Visible")
            n204 = local read "Camera Settings"() -> (w309:T2)
            n205 = Index Array(array=w310) -> (element=w313:cluster{string[]})  [unwired: 1 in]
            n206 = Unbundle(w309) -> ("Frame Rate"=w308:i32, "Compression"=w307:i32, "Size"=w311:u16)
            n207 = Unbundle(w313) -> (w312:string[])
            n208 = Index Array(array=w312, index=w311) -> (element=w306:string)
            n209 = call-poly <vilib>:"Write Key.vi"("section"=w317, "value"=w306, "key"="Size", "refnum"=w302) -> ("refnum out"=w319:T15)  [unwired: 2 in, 5 out]
            n210 = call-poly <vilib>:"Write Key.vi"("section"=w317, "value"=w308, "key"="FrameRate", "refnum"=w319) -> ("refnum out"=w318:T15)  [unwired: 1 in, 6 out]
            n211 = property on="Camera Settings" class="Clust (strict)"("Visible"=w320) -> ()  [unwired: 2 in, 2 out]
            n212 = local write "DB Camera Config"(w320) -> ()
            n213 = call-poly <vilib>:"Write Key.vi"("section"=w317, "value"=w307, "key"="Compression", "refnum"=w318) -> ("refnum out"=w304:T15)  [unwired: 1 in, 6 out]
            n214 = call <vilib>:"Close Config Data.vi"("refnum"=w304) -> ("file path"=w305:path)  [unwired: 2 in, 8 out]
            n215 = call <vilib>:"Open Config Data.vi"("configuration file path"=w305) -> ("refnum"=w303:T15)  [unwired: 8 in, 2 out]
          }
          frame True {
            n216 = property on="Camera Settings" class="Clust (strict)"("Visible"=TRUE) -> ()  [unwired: 2 in, 2 out]
          }
        }
      }
      event "Camera Settings": Value Change {
        # "Update summary string when any elements of DB camera change"
        n217 = event-data() -> ("NewVal"=w334:T2)  [unwired: 1 in]
        n218 = Index Array(array=w330) -> (element=w329:cluster{string[]})  [unwired: 1 in]
        n219 = Unbundle(w334) -> ("Frame Rate"=w325:i32, "Compression"=w324:i32, "Size"=w327:u16)
        n220 = Unbundle(w329) -> (w328:string[])
        n221 = Index Array(array=w328, index=w327) -> (element=w326:string)
        n222 = Format Into String(format string="%s   %dfps   %d%%", w326, w325, w324) -> (resulting string=w331:string)  [unwired: 2 in, 1 out]
        n223 = Build Array(w331) -> (w332:string[])
        n224 = property on="DB Camera Config" class="Bool (strict)"("Strings [4]"=w332) -> ()  [unwired: 2 in, 2 out]
      }
      event "Motor.Enable": Value Change {
        # "When the test mode otor enable helper is set, update that\ntree row item's value"
        n225 = event-data() -> ("NewVal"=w340:bool)  [unwired: 1 in]
        n226 = Unbundle("Motor") -> ("Value"=w339:dbl)  [unwired: 1 out]
        n227 = Select(t=w339, s=w340, f=0.0) -> (s? t:f=w337:dbl)
        n228 = call <vilib>:"NT Write Number.vi"("Numeric"=w337, "Name"=w336) -> ()  [unwired: 9 in, 1 out]
      }
      event "Test Slider": Value Change {
        # "When the test mode slider helper is set, update that\ntree row item's value"
        n229 = event-data() -> ("NewVal"=w343:dbl)  [unwired: 1 in]
        n230 = call <vilib>:"NT Write Number.vi"("Numeric"=w343, "Name"=w344) -> ()  [unwired: 9 in, 1 out]
      }
      event "On/Off": Value Change {
        # "When the test mode on/off helper value is set, update that\ntree row item's value"
        n231 = event-data() -> ("NewVal"=w348:bool)  [unwired: 1 in]
        n232 = Boolean To (0,1)(Boolean=w348) -> (0, 1=w347:i16)
        n233 = call <vilib>:"NT Write Number.vi"("Numeric"=w347, "Name"=w346) -> ()  [unwired: 9 in, 1 out]
      }
      event "Rev/Fwd": Value Change {
        # "When the test mode helper value for relays is set, update that\ntree row item's value"
        n234 = event-data() -> ("NewVal.Forward"=w356:bool, "NewVal.Reverse"=w355:bool)  [unwired: 1 in]
        n235 = Boolean To (0,1)(Boolean=w356) -> (0, 1=w352:i16)
        n236 = Boolean To (0,1)(Boolean=w355) -> (0, 1=w354:i16)
        n237 = Negate(x=w354) -> (-x=w353:i16)
        n238 = Add(x=w352, y=w353) -> (x+y=w351:i16)
        n239 = call <vilib>:"NT Write Number.vi"("Numeric"=w351, "Name"=w350) -> ()  [unwired: 9 in, 1 out]
      }
      event "Test Ring": Value Change {
        # "When a test mode helper value is selected from the ring,\nset the tree item's variable to the string value"
        n240 = event-data() -> ("NewVal"=w360:u16)  [unwired: 1 in]
        n241 = property on="Test Ring" class="Ring (strict)"() -> ("Strings []"=w361:string[])  [unwired: 2 in, 2 out]
        n242 = Index Array(array=w361, index=w360) -> (element=w359:string)
        n243 = call <vilib>:"NT Write String.vi"("String"=w359, "Name"=w358) -> ()  [unwired: 9 in, 1 out]
      }
      event "Rec Mode": Value Change {
        # "Update globals for recording mode and path to read log from.\nClear when logging and let NetworkTables set path for vision to\nuse."
        n244 = event-data() -> ("NewVal"=w371:enum32{"Stop", "Record", "Playback"})  [unwired: 1 in]
        n245 = global write "WPI_DashboardLogging Global.vi" "Logging Filename"(path "") -> ()
        n246 = case shown="\"Playback\"" w371 {
          tunnel: w370 -> [_ w373 w381]
          tunnel: [_ _ w380] -> w367
          tunnel: [_ _ w379] -> _
          tunnel: w365 -> [_ _ w377]
          tunnel: cluster{i32, i32} {-250, 170} -> [_ _ w376]
          tunnel: [_ _ T18 {"Image Size"=TRUE, "Image Type"=TRUE, "Pixel Value"=TRUE, "ROI Information"=TRUE, "Zoom Factor"=FALSE} ("Image Information Shown:All Elements")] -> w363
          tunnel: [_ _ TRUE ("Zoom Factor")] -> w362
          frame Default {
          }
          frame "Stop", "Record" {
            # "Place Window too"
            n247 = invoke class="VI" method="FP.Close"(reference=w373) -> (reference out=w372:refnum<vi>)  [unwired: 2 in, 2 out]
            n248 = invoke class="VI" method="Abort VI"(reference=w372) -> ()  [unwired: 2 in, 3 out]
          }
          frame "Playback" {
            n249 = call "Open Playback Panel.vi"("Offset"=w376, "DB VI Ref"=w377, "Playback in"=w381) -> ("Playback out"=w378:refnum<vi>)  [unwired: 8 in]
            n250 = register-events(w378) -> (reference out=w380:refnum<event-registration>, error out=w379:errorcluster)  [unwired: 2 in]
          }
        }
        n251 = global write "WPI_DashboardLogging Global.vi" "Recording"(w371) -> ()
        n252 = property on="Camera Image" class="ImageControl"("Image Information Shown"=w363, "Image Information Visible"=w362) -> ()  [unwired: 2 in, 2 out]
        n253 = call <vilib>:"WPI_DashboardNT Log FieldName Cache.vi"("Operation"=enum16{"Lookup/Add", "Index", "Clear"}."Clear") -> ()  [unwired: 8 in, 3 out]
      }
      event Panel Close {
        w382 = enum32{"Stop", "Record", "Playback"}."Stop" ("Rec Mode")
        # "Playback window has been closed, abort"
        n254 = event-data() -> ()  [unwired: 1 in, 4 out]
        n255 = local write "Rec Mode"(w382) -> ()
        n256 = global write "WPI_DashboardLogging Global.vi" "Recording"(w382) -> ()
      }
      event Panel Close {
        # "Abort playback window and ourself"
        n257 = event-data() -> ()  [unwired: 1 in, 4 out]
        n258 = invoke class="VI" method="FP.Close"(reference=w387) -> (reference out=w386:refnum<vi>)  [unwired: 2 in, 2 out]
        n259 = invoke class="VI" method="Abort VI"(reference=w386) -> (error out=w385:errorcluster)  [unwired: 2 in, 2 out]
        n260 = invoke class="VI" method="Abort VI"(error in=w385) -> ()  [unwired: 2 in, 3 out]
      }
      event "Vision": Value Change {
        # "Enable/Disable Compression slider.\nHW USB is hard-coded into the camera"
        n261 = event-data() -> ("NewVal"=w393:u16)  [unwired: 1 in]
        n262 = Equal?(x=w393, y=u32 2 ("milliseconds to wait")) -> (x = y?=w391:bool)
        n263 = Select(t=T19."Disabled and Grayed Out" ("Disabled"), s=w391, f=T19."Enabled" ("Disabled")) -> (s? t:f=w388:T19)
        n264 = property on="Compression" class="Slide (strict)"("DisabledEnum"=w388) -> ()  [unwired: 2 in, 2 out]
      }
    }
  }
  n265 = while {
    tunnel: w38 -> [w396]
    i -> [w399]
    stop <- FALSE stop-if-true
    n266 = Wait (ms)(milliseconds to wait=u32 100) -> ()  [unwired: 1 out]
    n267 = case shown="\"Playback\"" "Rec Mode" {
      tunnel: w399 -> [_ _ w414]
      tunnel: [u32 2829099 ("Base Color") u32 11141120 ("Target Color") w403] -> w395
      frame "Stop", Default {
        # "Reset the color, extra updates don't cost much"
      }
      frame "Record" {
      }
      frame "Playback" {
        # "Playback"
        n268 = Quotient & Remainder(x=w414, y=u32 50 ("milliseconds to wait")) -> (x-y*floor(x/y)=w410:u32)  [unwired: 1 out]
        n269 = Divide(x=w410, y=u32 50 ("milliseconds to wait")) -> (x/y=w407:dbl)
        n270 = Multiply(x=6.283185307179586, y=w407) -> (x*y=w412:dbl)
        n271 = Sine(x=w412) -> (sin(x)=w411:dbl)
        n272 = Absolute Value(x=w411) -> (abs(x)=w404:dbl)
        n273 = call "Interpolate RGB Color.vi"("Proportion"=w404, "Target Color"=u32 30976, "Base Color"=u32 2829099) -> ("Result Color"=w403:u32)  [unwired: 8 in]
      }
    }
    n274 = property class="Pane"(reference=w396, "PaneColor"=w395) -> ()  [unwired: 1 in, 2 out]
  }
  n275 = TCP Create Listener(10:u16 1741 ("timeout ms (25000)")) -> (3:w1:refnum<k5>)  [unwired: 4 in, 2 out]
  n276 = while {
    tunnel: w1 -> [w416]
    stop <- FALSE stop-if-true
    n277 = TCP Wait On Listener(11:w416) -> (4:w415:refnum<k5>)  [unwired: 3 in, 4 out]
    n278 = local write "TCP"(w415) -> ()
  }
  n279 = property on="On/Off" class="Bool (strict)"("Visible"=w6) -> ()  [unwired: 2 in, 2 out]
  n280 = property on="Motor" class="Clust (strict)"("Visible"=w6) -> ()  [unwired: 2 in, 2 out]
  n281 = property on="Progress" class="Clust (strict)"("Visible"=w6) -> ()  [unwired: 2 in, 2 out]
  n282 = property on="Test Ring" class="Ring (strict)"("Visible"=w6) -> ()  [unwired: 2 in, 2 out]
  n283 = property on="Rev/Fwd" class="Clust (strict)"("Visible"=w6) -> ()  [unwired: 2 in, 2 out]
  n284 = property on="Camera Settings" class="Clust (strict)"("Visible"=w6) -> ()  [unwired: 2 in, 2 out]
  n285 = local write "DB Camera Config"(w6) -> ()
  n286 = global write "WPI_DashboardLogging Global.vi" "Recording"(w32) -> ()
  n287 = local write "Rec Mode"(w32) -> ()
